vi "Configure Analog Gen Polarity.vi"(6 "Enable Waveform (T: Enable)":bool=TRUE, 7 "Frequency (10 Hz)":dbl=10.0, 8 "error in (no error)":errorcluster, 9 "Amplitude (0 Vrms)":dbl, 10 "Channel (0: A)":i32(ring) items=["A", "B"], 11 "VISA resource name":refnum<visa-resource-name>) -> (0 "error out":errorcluster, 3 "VISA resource name out":refnum<visa-resource-name>)   [LabVIEW 2014, in "Stanford Research SR1.lvlib"]
doc: "Configures the attributes for the Analog Generator Polarity."
uses:
  Stanford Research SR1.lvlib
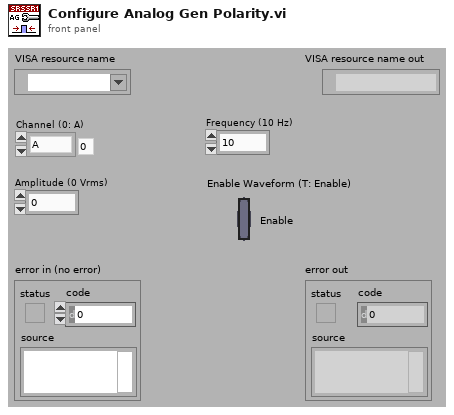
[diagram p1: front panel]
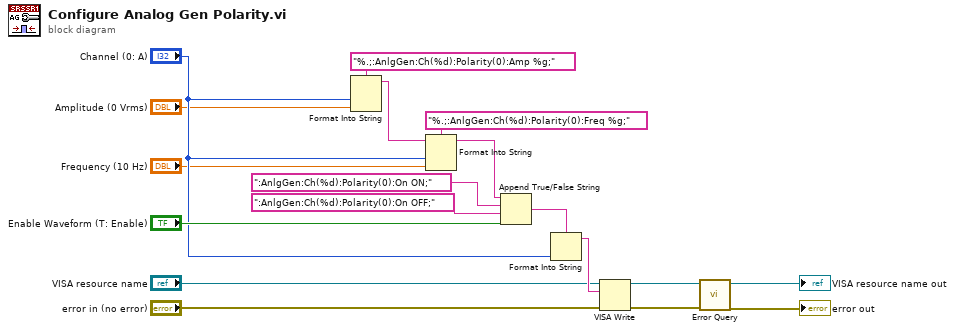
[diagram p0: block diagram]
diagram:
  n1 = Format Into String(format string="%.;:AnlgGen:Ch(%d):Polarity(0):Amp %g;", "Channel (0: A)", "Amplitude (0 Vrms)") -> (resulting string=w17:string)  [unwired: 2 in, 1 out]
  n2 = Format Into String(format string="%.;:AnlgGen:Ch(%d):Polarity(0):Freq %g;", initial string=w17, "Channel (0: A)", "Frequency (10 Hz)") -> (resulting string=w15:string)  [unwired: 1 in, 1 out]
  n3 = Append True/False String(1:"Enable Waveform (T: Enable)", 2:":AnlgGen:Ch(%d):Polarity(0):On OFF;", 3:":AnlgGen:Ch(%d):Polarity(0):On ON;", 4:w15) -> (0:w6:string)
  n4 = Format Into String(format string=w6, "Channel (0: A)") -> (resulting string=w5:string)  [unwired: 2 in, 1 out]
  n5 = VISA Write(VISA resource name="VISA resource name", write buffer=w5, error in (no error)="error in (no error)") -> (VISA resource name out=w10:refnum<visa-resource-name>, error out=w9:errorcluster)  [unwired: 1 out]
  n6 = call "Error Query.vi"("error in (no error)"=w9, "VISA resource name"=w10) -> ("error out"=→"error out":errorcluster, "VISA resource name out"=→"VISA resource name out":refnum<visa-resource-name>)  [unwired: 6 in, 2 out]
